vi "Withrawal MSG.vi"(8 "error in":errorcluster, 10 "variant":variant, 11 "ATM Data":T1) -> (0 "error out":errorcluster, 3 "ATM Data Out":T1)   [LabVIEW 2020]
uses:
  Cluster - ATM Machine Data.ctl
  Users/khemr/OneDrive/Desktop/Labview Training/CLD/New ATM_KR/ATM Machine/Cluster - Message Cluster.ctl
  Enum - ATM States.ctl
  98e35c26-2ff4-4b69-a813-136909b321a2.vi
  <vilib>/Comparison/Equal/Equal Functor/Equal Functor.lvclass
  ATM Machine.lvlib
panel:
  out "element":string
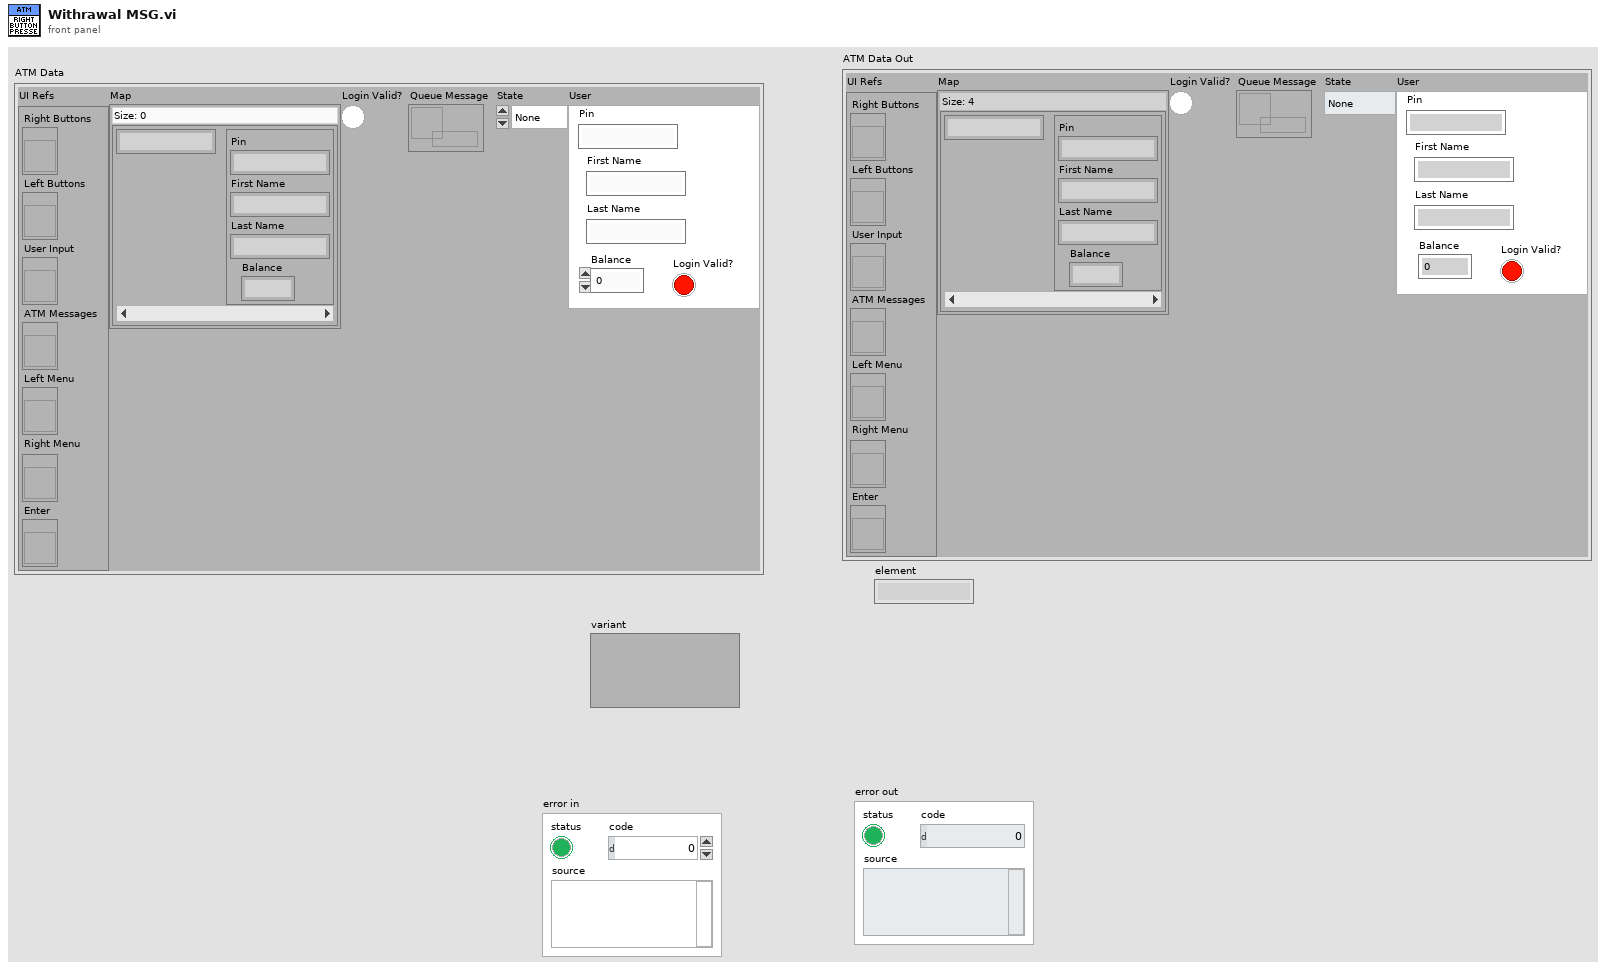
[diagram p1: front panel]
types:
  T1 = typedef "ATM Machine.lvlib/Cluster - ATM Machine Data.ctl" = cluster{"UI Refs":cluster{"Right Buttons":refnum<vi>, "Left Buttons":refnum<vi>, "User Input":refnum<vi>, "ATM Messages":refnum<vi>, "Left Menu":refnum<vi>, "Right Menu":refnum<vi>, "Enter":refnum<vi>}, "Map":map{string, cluster{"Pin":string, "First Name":string, "Last Name":string, "Balance":dbl}}, "Login Valid?":bool, "Queue Message":refnum<queue>, "State":T2, "User":cluster{"Pin":string, "First Name":string, "Last Name":string, "Balance":dbl, "Login Valid?":bool}}
  T2 = typedef "ATM Machine.lvlib/Enum - ATM States.ctl" = enum16{"None", "Deposit", "Withdraw", "Card Inserted", "Balance Inquiry", "Return Card and Terminate", "Fast Cash"}
  T3 = cluster{"RFS String":string, "RFS String 2":string, "RFS String 3":string}
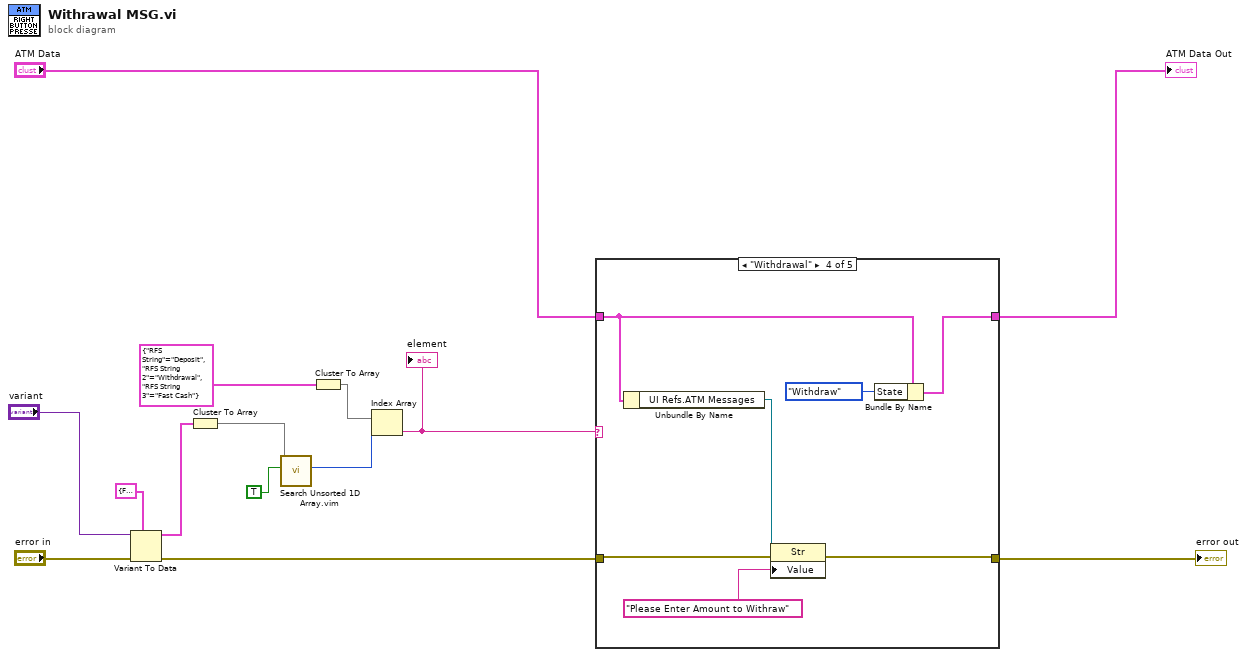
[diagram p0: block diagram]
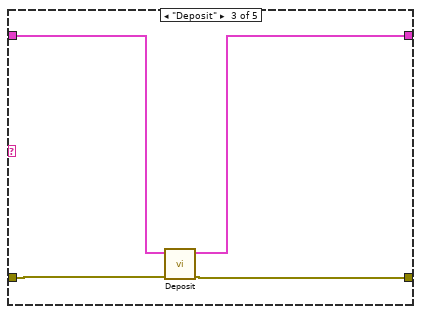
[diagram p4: hidden frame]
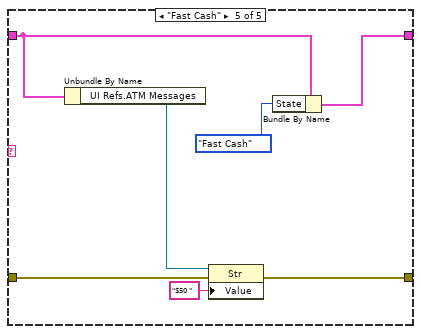
[diagram p5: hidden frame]
diagram:
  n1 = Variant To Data(error in="error in", type=cluster{bool, bool, bool} {FALSE, FALSE, FALSE}, Variant="variant") -> (data=w11:cluster{bool, bool, bool}, error out=w1:errorcluster)
  n2 = Cluster To Array(cluster=w11) -> (array=w10:bool[])
  n3 = call "Search Unsorted 1D Array.vim"("element"=TRUE, "unsorted 1D array"=w10) -> ("index of element"=w7:i32)  [unwired: 9 in]
  n4 = Cluster To Array(cluster=T3 {"RFS String"="Deposit", "RFS String 2"="Withdrawal", "RFS String 3"="Fast Cash"} ("Right Menu")) -> (array=w8:string[])
  n5 = Index Array(array=w8, index=w7) -> (element=w5:string)
  "element" <- w5
  n6 = case shown="\"Withdrawal\"" w5 {
    tunnel: "ATM Data" -> [w16 w18 w20 w23 w30]
    tunnel: [w16 w18 w19 w24 w31] -> w3
    tunnel: [w15 w17 w21 w28 w35] -> w2
    tunnel: w1 -> [w15 w17 w22 w29 w36]
    frame "False", Default {
    }
    frame "True" {
    }
    frame "Deposit" {
      n7 = call "Deposit.vi"("error in"=w22, "ATM Data"=w20) -> ("error out"=w21:errorcluster, "ATM Data Out"=w19:T1)  [unwired: 8 in]
    }
    frame "Withdrawal" {
      n8 = Unbundle By Name(w23) -> ("UI Refs.ATM Messages"=w27:refnum<vi>)
      n9 = property class="Str"(reference=w27, error in=w29, "Value"="Please Enter Amount to Withraw") -> (error out=w28:errorcluster)  [unwired: 1 out]
      n10 = Bundle By Name(cluster=w23, "State"=Enum_-_ATM_States."Withdraw") -> (w24:T1)
    }
    frame "Fast Cash" {
      n11 = Unbundle By Name(w30) -> ("UI Refs.ATM Messages"=w34:refnum<vi>)
      n12 = property class="Str"(reference=w34, error in=w36, "Value"="$50 ") -> (error out=w35:errorcluster)  [unwired: 1 out]
      n13 = Bundle By Name(cluster=w30, "State"=Enum_-_ATM_States."Fast Cash") -> (w31:T1)
    }
  }
  "ATM Data Out" <- w3
  "error out" <- w2
